vi "Forward Kinematics.vi"(6 "L(m)":dbl, 8 "r(m)":dbl, 9 "Phi3(rad/s)":dbl, 10 "Phi2(rad/s)":dbl, 11 "Phi1(rad/s)":dbl) -> (1 "Theta(deg/s)":dbl, 2 "Y(m/s)":dbl, 3 "X(m/s)":dbl)   [LabVIEW 2019]
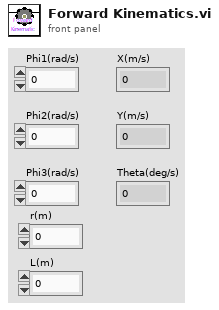
[diagram p1: front panel]
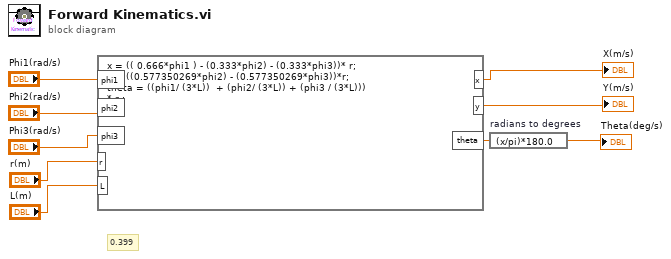
[diagram p0: block diagram]
diagram:
  # "0.399"
  n1 = formula code="x = (( 0.666*phi1 ) - (0.333*phi2) - (0.333*phi3))* r;\ny = ((0.577350269*phi2) - (0.577350269*phi3))*r;\ntheta = ((phi1/ (3*L))  + (phi2/ (3*L)) + (phi3 / (3*L))) \n* r ;"("phi1"="Phi1(rad/s)", "phi2"="Phi2(rad/s)", "phi3"="Phi3(rad/s)", "r"="r(m)", "L"="L(m)") -> ("x"=→"X(m/s)":dbl, "y"=→"Y(m/s)":dbl, "theta"=w3:dbl)
  n2 = expression code="(x/pi)*180.0" "radians to degrees"(w3) -> (→"Theta(deg/s)":dbl)
